vi "Send Control Drag Over.vi"(0 "Message Enqueuer in":refnum<class "Message Enqueuer.lvclass">, 3 "EventFilter Reference":T2, 5 "CtlRef":refnum<vi>, 7 "Time":u32, 9 "Coords":T1, 11 "Button":u16, 12 "Mods":cluster{"Double Click":bool, "Menu Key":bool}, 13 "PlatMods":T3, 14 "Available Data Names":string[](array[string])) -> (4 "Filtered EventDataMessage":refnum<class "ControlDragOverMsg.lvclass">, 15 "error out":errorcluster)   [LabVIEW 2015, in "ActorEvents.lvlib" / "ControlDragOverMsg.lvclass"]
doc: "<License>\nCopyright © 2017 Composed Systems, LLC | All rights reserved\nwww.composed.io\n\nAuthor: Ethan Stern <ethan.stern@composed.io>\n\nThis software is provided \"AS IS\" WITHOUT WARRANTIES, either express or implied, AND IS FOR EDUCATIONAL PURPOSES ONLY.\n</License>"
uses:
  ControlDragOverMsg.lvclass
  <vilib>/ActorFramework/Message Enqueuer/Message Enqueuer.lvclass
  IEventFilter/EventFilter Reference.ctl
  IEventFilter/IEventFilter.lvclass
  <vilib>/Utility/miscctls.llb/LVPoint32TypeDef.ctl
  ControlDragOverMsg.lvclass/ControlDragOverMsg.ctl
  EventDataMessage/EventDataMessage.lvclass/EventDataMessage.ctl
  <vilib>/ActorFramework/Message Enqueuer/Message Enqueuer.lvclass/Message Enqueuer.ctl
  <vilib>/ActorFramework/Message Enqueuer/Enqueue.vi
  <vilib>/Utility/error.llb/Clear Errors.vi
  <vilib>/ActorFramework/Message Priority Queue/Priority Enqueue.vi
  EventDataMessage/EventDataMessage.lvclass
panel:
  in  "error in (no error)":errorcluster
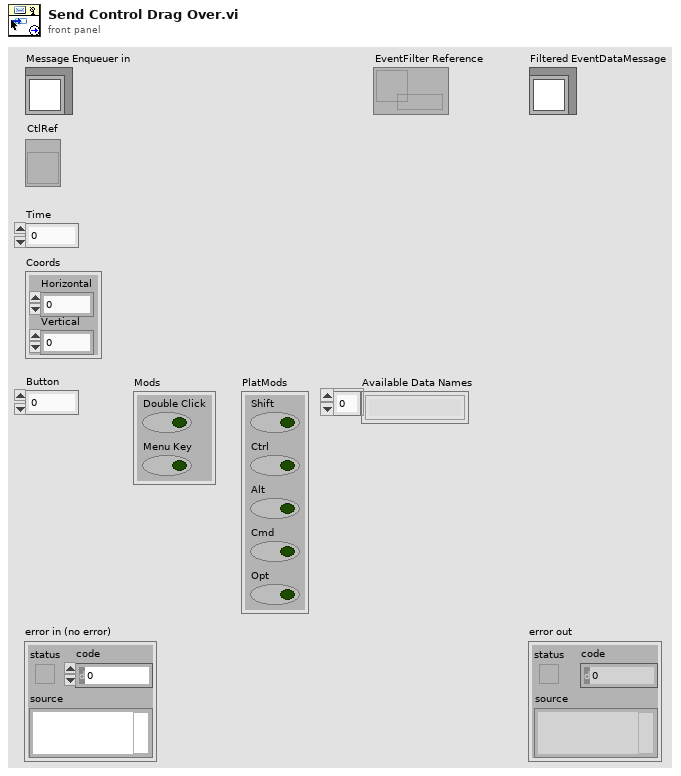
[diagram p1: front panel]
types:
  T1 = typedef "LVPoint32TypeDef.ctl" = cluster{"Horizontal":i32, "Vertical":i32}
  T2 = typedef "ActorEvents.lvlib/IEventFilter.lvclass/EventFilter Reference.ctl" = refnum<data-value>
  T3 = cluster{"Shift":bool, "Ctrl":bool, "Alt":bool, "Cmd":bool, "Opt":bool}
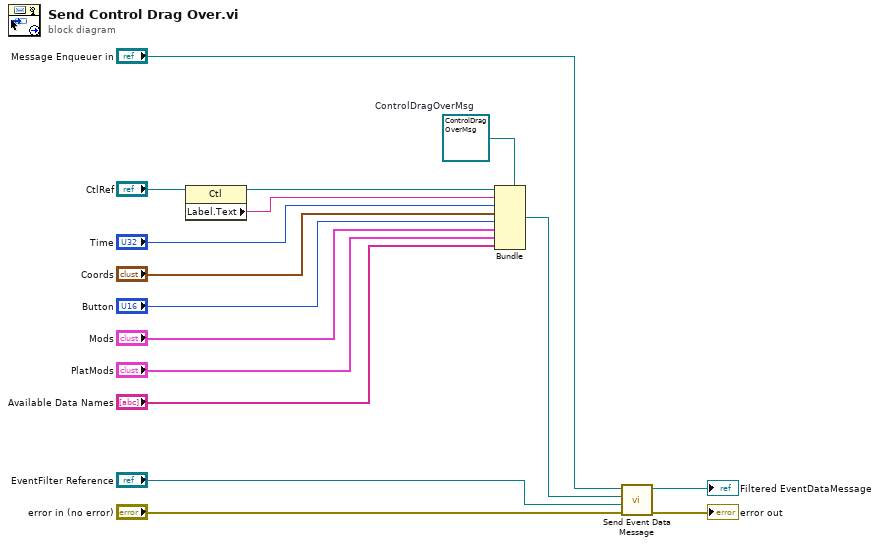
[diagram p0: block diagram]
diagram:
  w16 = refnum<class "ControlDragOverMsg.lvclass"> refnum  # ControlDragOverMsg
  n1 = property class="Ctl"(reference="CtlRef") -> (reference out=w10:refnum<vi>, "Label.Text"=w9:string)  [unwired: 1 in, 1 out]
  n2 = Bundle(cluster=w16, w10, w9, "Time", "Coords", "Button", "Mods", "PlatMods", "Available Data Names") -> (w13:refnum<class "ControlDragOverMsg.lvclass">)
  n3 = call "Send Event Data Message.vi"("error in (no error)"="error in (no error)", "EventFilter Reference"="EventFilter Reference", "EventDataMessage"=w13, "Message Enqueuer in"="Message Enqueuer in") -> ("error out"=→"error out":errorcluster, "Filtered EventDataMessage"=→"Filtered EventDataMessage":refnum<class "ControlDragOverMsg.lvclass">)  [unwired: 6 in]
